vi "7.5.vi"() -> ()   [LabVIEW 2017]
uses:
  <vilib>/measure/NI_MABase.lvlib
panel:
  in  "停止":bool
  in  "可见":bool
  out "波形图":waveform(dbl)(graph)
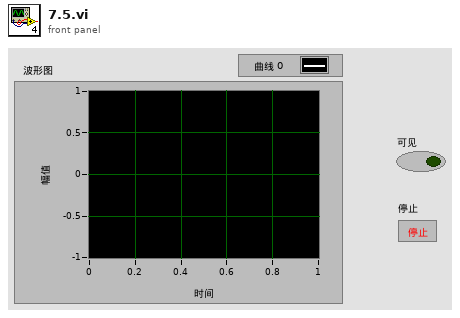
[diagram p1: front panel]
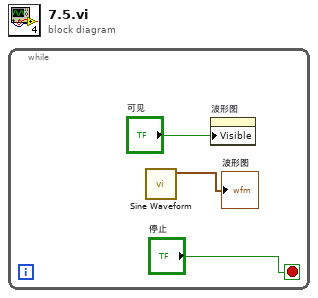
[diagram p0: block diagram]
diagram:
  n1 = while {
    stop <- "停止" stop-if-true
    n2 = call <vilib>:"Sine Waveform.vi"() -> ("signal out"=→"波形图":waveform(dbl))  [unwired: 10 in, 1 out]
    n3 = property on="波形图" class="WFGraph (严格)"("Visible"="可见") -> ()  [unwired: 2 in, 2 out]
  }
